vi "Jenkins Build Done.vi"(8 "error in (no error)":errorcluster, 10 "Build Error":errorcluster, 11 "Project Builder in":refnum<class "Project Builder.lvclass">) -> (0 "error out":errorcluster, 3 "Project Builder out":refnum<class "Project Builder.lvclass">)   [LabVIEW 2014, in "Project Builder.lvclass"]
uses:
  Project Builder.lvclass
  Project Builder.lvclass/Project Builder.ctl
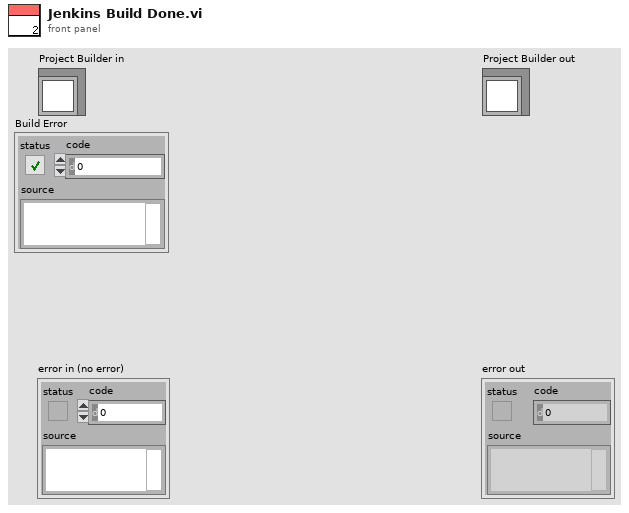
[diagram p1: front panel]
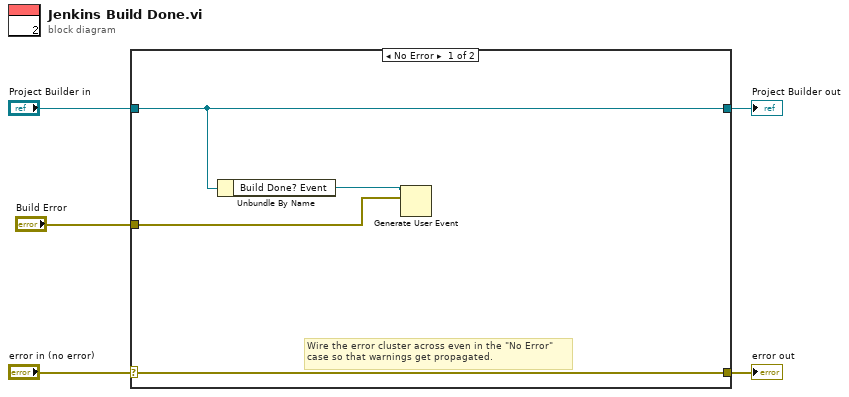
[diagram p0: block diagram]
diagram:
  n1 = case shown="No Error" "error in (no error)" {
    selector: "error in (no error)" -> [w9 w11]
    tunnel: [w9 w11] -> w4
    tunnel: [w8 w10] -> w2
    tunnel: "Project Builder in" -> [w8 w10]
    tunnel: "Build Error" -> [w6 _]
    frame No Error {
      # "Wire the error cluster across even in the \"No Error\"\ncase so that warnings get propagated."
      n2 = Unbundle By Name(w8) -> ("Build Done? Event"=w7:refnum<user-event>)
      n3 = Generate User Event(user event=w7, event data cluster=w6) -> ()  [unwired: 2 in, 2 out]
    }
    frame Error {
    }
  }
  "error out" <- w4
  "Project Builder out" <- w2
